vi "niDTS WLAN Tx Test Full Example.vi"() -> ()   [LabVIEW 2014]
uses:
  CommLib/Includes/niDTS Comm INC Telnet Port Parameters.ctl
  CommLib/Includes/niDTS Comm INC CLI Login.ctl
  CommLib/Includes/niDTS Comm INC EXE Port Parameters.ctl
  Includes/niDTS WLAN INC Type.ctl
  OFDM Tx Test/Includes/niDTS WLAN OFDM Tx Test INC Parameters.ctl
  Includes/niDTS WLAN INC OFDM Data Rate.ctl
  Includes/niDTS WLAN INC CH BW DSSS.ctl
  Includes/niDTS WLAN DUT INC Acquisition Parameters.ctl
  Includes/niDTS WLAN INC TXP Measurement Parameters.ctl
  OFDM Tx Test/Includes/niDTS WLAN OFDM Tx Test INC ModAcc Measurement Parameters.ctl
  Includes/niDTS WLAN INC SEM Measurement Parameters.ctl
  Includes/niDTS WLAN INC OBW Measurement Parameters.ctl
  HT Tx Test/Includes/niDTS WLAN HT Tx Test INC Parameters.ctl
  Includes/niDTS WLAN INC CH BW HT.ctl
  Includes/niDTS WLAN INC GI.ctl
  Includes/niDTS WLAN INC FEC Coding.ctl
  VHT Tx Test/Includes/niDTS WLAN VHT Tx Test INC Parameters.ctl
  Includes/niDTS WLAN INC CH BW.ctl
  Tx Test/Includes/niDTS WLAN Tx Test INC Results.ctl
  Tx Test/Includes/niDTS WLAN Tx Test INC MOD EVM Results.ctl
  Tx Test/Includes/Results/niDTS Tx RES INC EVM.ctl
  Tx Test/Includes/niDTS WLAN Tx Test INC TXP Results.ctl
  Tx Test/Includes/niDTS WLAN Tx Test INC TXP Result SINGLE.ctl
  Tx Test/Includes/niDTS WLAN Tx Test INC OBW Results.ctl
  Instrument/INSTR TX/Results/niDTS WLAN INSTR TX INC SEM Results.ctl
  Instrument/INSTR TX/Results/niDTS WLAN INSTR TX INC SEM FSEGemts Results.ctl
  Tx Test/Includes/Results/niDTS Tx RES INC SEM FSEGemts.ctl
  Instrument/INSTR TX/Results/niDTS WLAN INSTR TX INC SEM MARGin Results.ctl
  Tx Test/Includes/Results/niDTS Tx RES INC SEM Margin.ctl
  Instrument/INSTR TX/Results/niDTS WLAN INSTR TX INC OFDM Impairments Results.ctl
  DSSS Tx Test/Includes/niDTS WLAN DSSS Tx Test INC Parameters.ctl
  Includes/niDTS WLAN INC DSSS Data Rate.ctl
  Includes/niDTS WLAN INC Channel DSSS.ctl
  DSSS Tx Test/Includes/niDTS WLAN DSSS Tx Test INC ModAcc Measurement Parameters.ctl
  Includes/niDTS WLAN INC Pulse Shaping Filter Type.ctl
  Includes/niDTS WLAN INC DSSS Power Ramp Parameters.ctl
  Tx Test/Includes/niDTS WLAN Tx Test INC DSSS Results.ctl
  Tx Test/Includes/niDTS WLAN Tx Test INC DSSS MOD EVM Results.ctl
  DSSS Tx Test/Includes/Results/niDTS WLAN DSSS Tx RES EVM ALL.ctl
  DSSS Tx Test/Includes/Results/niDTS WLAN DSSS Tx RES EVM RMS.ctl
  Tx Test/Includes/niDTS WLAN Tx Test INC DSSS MOD Impairments Results.ctl
  DSSS Tx Test/Includes/Results/niDTS WLAN DSSS Tx Impairmentsctl.ctl
  DSSS Tx Test/Includes/Results/niDTS WLAN DSSS Tx PowerRamp.ctl
  TestStand/Station/Objects/SystemDutHandle/niDTS SystemDutHandle.lvclass
  niDTS WLAN.lvlib
  Framework/niDTS Framework.lvlib
  TestStand/niDTS TestStand.lvlib
  Plugins/niBCM4360/niBCM4360.lvlib
  Plugins/niBCM4350/niBCM4350.lvlib
  Plugins/niWTM Loopback/niWTM Loopback.lvlib
  CommLib/niDTS CommLib.lvlib
  Plugins/niBCM4356/niBCM4356.lvlib
  Framework/Logger/Listener/Viewer/niDTS Logger Listener Viewer.lvclass
  Instrument/INSTR TX/niDTS WLAN INSTR TX.lvclass
panel:
  in  "Keep Log Open":bool
  out "DSSS Results":T1 {"OBW"."Stop Frequency (Hz)" format="%#_4p"; "OBW"."Start Frequency (Hz)" format="%#_4p"; "OBW"."OBW (Hz)" format="%#_4p"}
  in  "ResultsIndex":u8=1
  in  "System Configuration XML Path":path=path "C:/Users/Public/Documents/National Instruments/WTM 1.0/System Configurations"
  in  "Socket Index":i32
  out "Results":T16={"Stream ModAcc"={"EVM"={"OFDM EVM Average"=[{"Stream Index"=1, "Packet (dB)"=-38.670074, "Pilot (dB)"=-40.331799, "Data (dB)"=-38.562389}], "OFDM EVM Max"=[{"Stream Index"=1, "Packet (dB)"=-38.670074, "Pilot (dB)"=-40.331799, "Data (dB)"=-38.562389}], "OFDM EVM Min"=[{"Stream Index"=1, "Packet (dB)"=-38.670074, "Pilot (dB)"=-40.331799, "Data (dB)"=-38.562389}]}}, "Channel ModAcc"={"EVM"={"OFDM EVM Average"=[{"Stream Index"=1, "Packet (dB)"=-38.670074, "Pilot (dB)"=-40.331799, "Data (dB)"=-38.562389}], "OFDM EVM Max"=[{"Stream Index"=1, "Packet (dB)"=-38.670074, "Pilot (dB)"=-40.331799, "Data (dB)"=-38.562389}], "OFDM EVM Min"=[{"Stream Index"=1, "Packet (dB)"=-38.670074, "Pilot (dB)"=-40.331799, "Data (dB)"=-38.562389}]}}, "TXP"={"Average"=[{"Chain Index"=1.0, "Average Power (dBm)"=-12.457251, "Peak Power (dBm)"=-4.586085, "Avg Power w Gap (dBm)"=-12.457251}], "Max"=[{"Chain Index"=1.0, "Average Power (dBm)"=-12.457251, "Peak Power (dBm)"=-4.586085, "Avg Power w Gap (dBm)"=-12.457251}], "Min"=[{"Chain Index"=1.0, "Average Power (dBm)"=-12.457251, "Peak Power (dBm)"=-4.586085, "Avg Power w Gap (dBm)"=-12.457251}]}, "OBW"=[{"Chain Index"=1.0, "OBW (Hz)"=17635824.926234, "Start Frequency (Hz)"=5171217983.349262, "Stop Frequency (Hz)"=5188853808.275496}], "SEM Results"={"SEM:FSEGemts"=[], "Margin"=[{"Chain Index"=1, "Worst Case Out Of Band Margin (dB)"=7.826486, "Worst Case Out Of Band Frequency (Hz)"=5191096938.77551, "Violation (%)"=0.0}]}, "OFDM Impairments"={"Average"={"Sample Clock Offset (ppm)"=1.406776, "Carrier Frequency Offset (ppm)"=19.372688, "Avg Rms Com Pilot Error (%)"=0.861502, "Rms Phase Noise (deg)"=0.437853, "ChannelData"=[{"Channel Index"=1, "IQ Imbalance (dB)"=0.0028770000000000002, "Quadrature Skew (deg)"=0.012293, "Carrier Leakage (dB)"=-55.264069, "Timing Skew (s)"=0.0}]}, "Max"={"Sample Clock Offset (ppm)"=1.406776, "Carrier Frequency Offset (ppm)"=19.372688, "Avg Rms Com Pilot Error (%)"=0.861502, "Rms Phase Noise (deg)"=0.437853, "ChannelData"=[{"Channel Index"=1, "IQ Imbalance (dB)"=0.0028770000000000002, "Quadrature Skew (deg)"=0.012293, "Carrier Leakage (dB)"=-55.264069, "Timing Skew (s)"=0.0}]}, "Min"={"Sample Clock Offset (ppm)"=1.406776, "Carrier Frequency Offset (ppm)"=19.372688, "Avg Rms Com Pilot Error (%)"=0.861502, "Rms Phase Noise (deg)"=0.437853, "ChannelData"=[{"Channel Index"=1, "IQ Imbalance (dB)"=0.0028770000000000002, "Quadrature Skew (deg)"=0.012293, "Carrier Leakage (dB)"=-55.264069, "Timing Skew (s)"=0.0}]}}} {"OBW"."Stop Frequency (Hz)" format="%#_4p"; "OBW"."Start Frequency (Hz)" format="%#_4p"; "OBW"."OBW (Hz)" format="%#_4p"}
  out "error out":errorcluster
  in  "DUT Plugin":T20(tab)=enum."BCM4356"
  in  "Interfaces BCM4350":enum32{".EXE", "Telnet"}(tab)
  in  "General Parameters bcm4350 exe":T22={"WLAN"={"Port Parameters EXE"={"Timeout (s)"=5.0}}} caption="General Parameters"
  in  "Socket Parameters bcm4350 exe":cluster{"WLAN":cluster{"IP Address":string}}={"WLAN"={"IP Address"="192.168.1.1"}} caption="Socket Parameters"
  in  "Socket Parameters bcm4350 telnet":cluster{"WLAN":cluster{"IP Address":string}}={"WLAN"={"IP Address"="192.168.1.1"}} caption="Socket Parameters"
  in  "General Parameters bcm4350 telnet":T25={"WLAN"={"Port Parameters Telnet"={"Bytes to Read"=1000, "Line Separator"="\n", "Port Timeout (ms)"=5000, "Read Mode"=enum."normal", "Write Mode"=enum."normal", "Remote Port"=23}, "CLI Login"={"Do Login"=FALSE, "Login Prompt"="", "Password"="", "User Name"=""}}} caption="General Parameters"
  in  "General Parameters 4":T25={"WLAN"={"Port Parameters Telnet"={"Bytes to Read"=1000, "Line Separator"="\n", "Port Timeout (ms)"=5000, "Read Mode"=enum."normal", "Write Mode"=enum."normal", "Remote Port"=23}, "CLI Login"={"Do Login"=TRUE, "Login Prompt"="localhost login: ", "Password"="labview", "User Name"="root"}}} caption="General Parameters"
  in  "Socket Parameters bcm4356":cluster{"WLAN":cluster{"IP Address":string}}[](array[cluster])=[{"WLAN"={"IP Address"="192.168.0.31"}}, {"WLAN"={"IP Address"="192.168.0.32"}}, {"WLAN"={"IP Address"="192.168.0.33"}}, {"WLAN"={"IP Address"="192.168.0.34"}}] caption="Socket Parameters"
  in  "Socket Parameters":T26={"WLAN"={"VISA Resource"="TCPIP0::InstrumentAddress::inst0::INSTR", "PortNames "=["Port0"]}}
  in  "General Parameters":T27={"WLAN"={"Idle Interval (s)"=0.0001, "Payload Length Limit (bytes)"=12000, "Channel Secondary Factor"=enum."0"}} {"WLAN"."Idle Interval (s)" format="%_3p"}
  in  "Test Config":enum32{"DSSS", "OFDM", "HT", "VHT"}(tab)=enum."OFDM"
  in  "DSSS Parameters":T28={"DSSS Data Rate (Mbps)"=enum."1", "Chains"=[TRUE, FALSE, FALSE, FALSE], "Bandwidth (Hz)"=enum."20 MHz", "Channel"=1, "Dut Tx Power  (dBm)"=-20.0, "16 symbols"=TRUE, "Payload Length (bytes)"=1500, "Idle Interval (s)"=0.0001, "External Attenuation (dB)"=[0.0, 0.0, 0.0, 0.0], "Acquisition "={"Acquisition Length Mode"=enum."AUTO", "Acquisition Length (s)"=0.00015, "Auto Level"=FALSE}, "TXP Measurement"={"TXP Power Enable"=TRUE, "TXP Averages"=1}, "ModAcc Measurement"={"ModAcc Enable"=TRUE, "Header Detection"=enum."FIRST", "Averages"=1, "CFO Estimation"=enum."PAMBLE", "DC Offset Compensation"=FALSE, "Chip Start Location"=0, "Max Chips Used"=16, "Pulse Shaping FilterType"=enum."RCOSINE", "Pulse Shaping Filter Coefficient"=0.35, "Equalization"=TRUE, "Phase Tracking"=TRUE}, "SEM Measurement"={"SEM Enable"=TRUE, "SEM Averages"=1, "Auto Span Enable"=TRUE, "Frequency Span (Hz)"=66000000.0, "Measurement Type"=enum."Standard", "Mask Frequencies (Hz)"=[], "Mask Power Offsets (dB)"=[]}, "OBW Measurement"={"OBW Enable"=TRUE, "OBW Averages"=1}, "DSSS Power Ramp"={"Power Ramp Enable"=TRUE, "Averages"=3, "Thresholds"={"Up Low (%)"=10.0, "Down Low (%)"=10.0, "Up High (%)"=90.0, "Down High (%)"=90.0}}} {"DSSS Power Ramp"."Thresholds"."Down High (%)" min=0.0 max=100.0 step=1.0; "DSSS Power Ramp"."Thresholds"."Up High (%)" min=0.0 max=100.0 step=1.0; "DSSS Power Ramp"."Thresholds"."Down Low (%)" min=0.0 max=100.0 step=1.0; "DSSS Power Ramp"."Thresholds"."Up Low (%)" min=0.0 max=100.0 step=1.0; "Acquisition"."Acquisition Length (s)" format="%#_6p"; "SEM Measurement"."Frequency Span (Hz)" format="%#_6p"; "Channel" items=["1"=1, "2"=2, "3"=3, "4"=4, "5"=5, "6"=6, "7"=7, "8"=8, "9"=9, "10"=10, "11"=11, "12"=12, "13"=13, "14"=14]; "Idle Interval (s)" format="%_3p"}
  in  "OFDM Parameters":T39={"OFDM Data Rate (Mbps)"=enum."54", "Chains"=[TRUE, FALSE, FALSE, FALSE], "Bandwidth (Hz)"=enum."20 MHz", "Channel"=36, "Dut Tx Power (dBm)"=-20.0, "16 symbols"=TRUE, "Payload Length (bytes)"=1500, "Idle Interval (s)"=0.0001, "External Attenuation (dB)"=[0.0, 0.0, 0.0, 0.0], "Acquisition "={"Acquisition Length Mode"=enum."AUTO", "Acquisition Length (s)"=0.00015, "Auto Level"=FALSE}, "TXP Measurement"={"TXP Power Enable"=TRUE, "TXP Averages"=1}, "ModAcc Measurement"={"ModAcc Enable"=TRUE, "Header Detection"=enum."FIRST", "Averages"=1, "CFO Estimation"=enum."PAMBLE", "Amplitude Tracking"=FALSE, "Channel Tracking"=FALSE, "Time Tracking"=TRUE, "Phase Tracking"=enum."STANDARD", "Clock Offset Est"=TRUE, "Impairments Est"=TRUE}, "SEM Measurement"={"SEM Enable"=TRUE, "SEM Averages"=1, "Auto Span Enable"=TRUE, "Frequency Span (Hz)"=66000000.0, "Measurement Type"=enum."Standard", "Mask Frequencies (Hz)"=[], "Mask Power Offsets (dB)"=[]}, "OBW Measurement"={"OBW Enable"=TRUE, "OBW Averages"=1}} {"Acquisition"."Acquisition Length (s)" format="%#_6p"; "SEM Measurement"."Frequency Span (Hz)" format="%#_6p"; "Idle Interval (s)" format="%_3p"}
  in  "HT Parameters":T42={"MCS Index"=7, "Chains"=[TRUE, FALSE, FALSE, FALSE], "Bandwidth (Hz)"=enum."20 MHz", "Channel"=36, "Gard Interval"=enum."LONG", "FEC Coding"=enum."LDPC", "Dut Tx Power (dBm)"=10.0, "16 symbols"=TRUE, "Payload Length (bytes)"=1500, "Idle Interval (s)"=0.0001, "External Attenuation (dB)"=[0.0, 0.0, 0.0, 0.0], "Acquisition"={"Acquisition Length Mode"=enum."AUTO", "Acquisition Length (s)"=0.00015, "Auto Level"=FALSE}, "TXP Measurement"={"TXP Power Enable"=TRUE, "TXP Averages"=1}, "ModAcc Measurement"={"ModAcc Enable"=TRUE, "Header Detection"=enum."FIRST", "Averages"=1, "CFO Estimation"=enum."PAMBLE", "Amplitude Tracking"=FALSE, "Channel Tracking"=FALSE, "Time Tracking"=TRUE, "Phase Tracking"=enum."STANDARD", "Clock Offset Est"=TRUE, "Impairments Est"=TRUE}, "SEM Measurement"={"SEM Enable"=TRUE, "SEM Averages"=1, "Auto Span Enable"=TRUE, "Frequency Span (Hz)"=66000000.0, "Measurement Type"=enum."Standard", "Mask Frequencies (Hz)"=[], "Mask Power Offsets (dB)"=[]}, "OBW Measurement"={"OBW Enable"=TRUE, "OBW Averages"=1}} {"Acquisition"."Acquisition Length (s)" format="%#_6p"; "SEM Measurement"."Frequency Span (Hz)" format="%#_6p"; "Idle Interval (s)" format="%_3p"}
  in  "VHT Parameters":T46={"MCS Index"=7, "N Spatial Streams"=1, "Chains"=[TRUE, FALSE, FALSE, FALSE], "Bandwidth (Hz)"=enum."20 MHz", "Channel"=36, "Gard Interval"=enum."LONG", "FEC Coding"=enum."LDPC", "Dut Tx Power (dBm)"=-20.0, "16 symbols"=TRUE, "Payload Length (bytes)"=1500, "Idle Interval (s)"=0.0001, "External Attenuation (dB)"=[0.0, 0.0, 0.0, 0.0], "Acquisition "={"Acquisition Length Mode"=enum."AUTO", "Acquisition Length (s)"=0.00015, "Auto Level"=FALSE}, "TXP Measurement"={"TXP Power Enable"=TRUE, "TXP Averages"=1}, "ModAcc Measurement"={"ModAcc Enable"=TRUE, "Header Detection"=enum."FIRST", "Averages"=1, "CFO Estimation"=enum."PAMBLE", "Amplitude Tracking"=FALSE, "Channel Tracking"=FALSE, "Time Tracking"=TRUE, "Phase Tracking"=enum."STANDARD", "Clock Offset Est"=TRUE, "Impairments Est"=TRUE}, "SEM Measurement"={"SEM Enable"=TRUE, "SEM Averages"=1, "Auto Span Enable"=TRUE, "Frequency Span (Hz)"=66000000.0, "Measurement Type"=enum."Standard", "Mask Frequencies (Hz)"=[], "Mask Power Offsets (dB)"=[]}, "OBW Measurement"={"OBW Enable"=TRUE, "OBW Averages"=1}} {"Acquisition"."Acquisition Length (s)" format="%#_6p"; "SEM Measurement"."Frequency Span (Hz)" format="%#_6p"; "Idle Interval (s)" format="%_3p"}
  out "Results Type":T48=enum."n - MCS7"
  # "No Options"
  # "Note the \\s after login:"
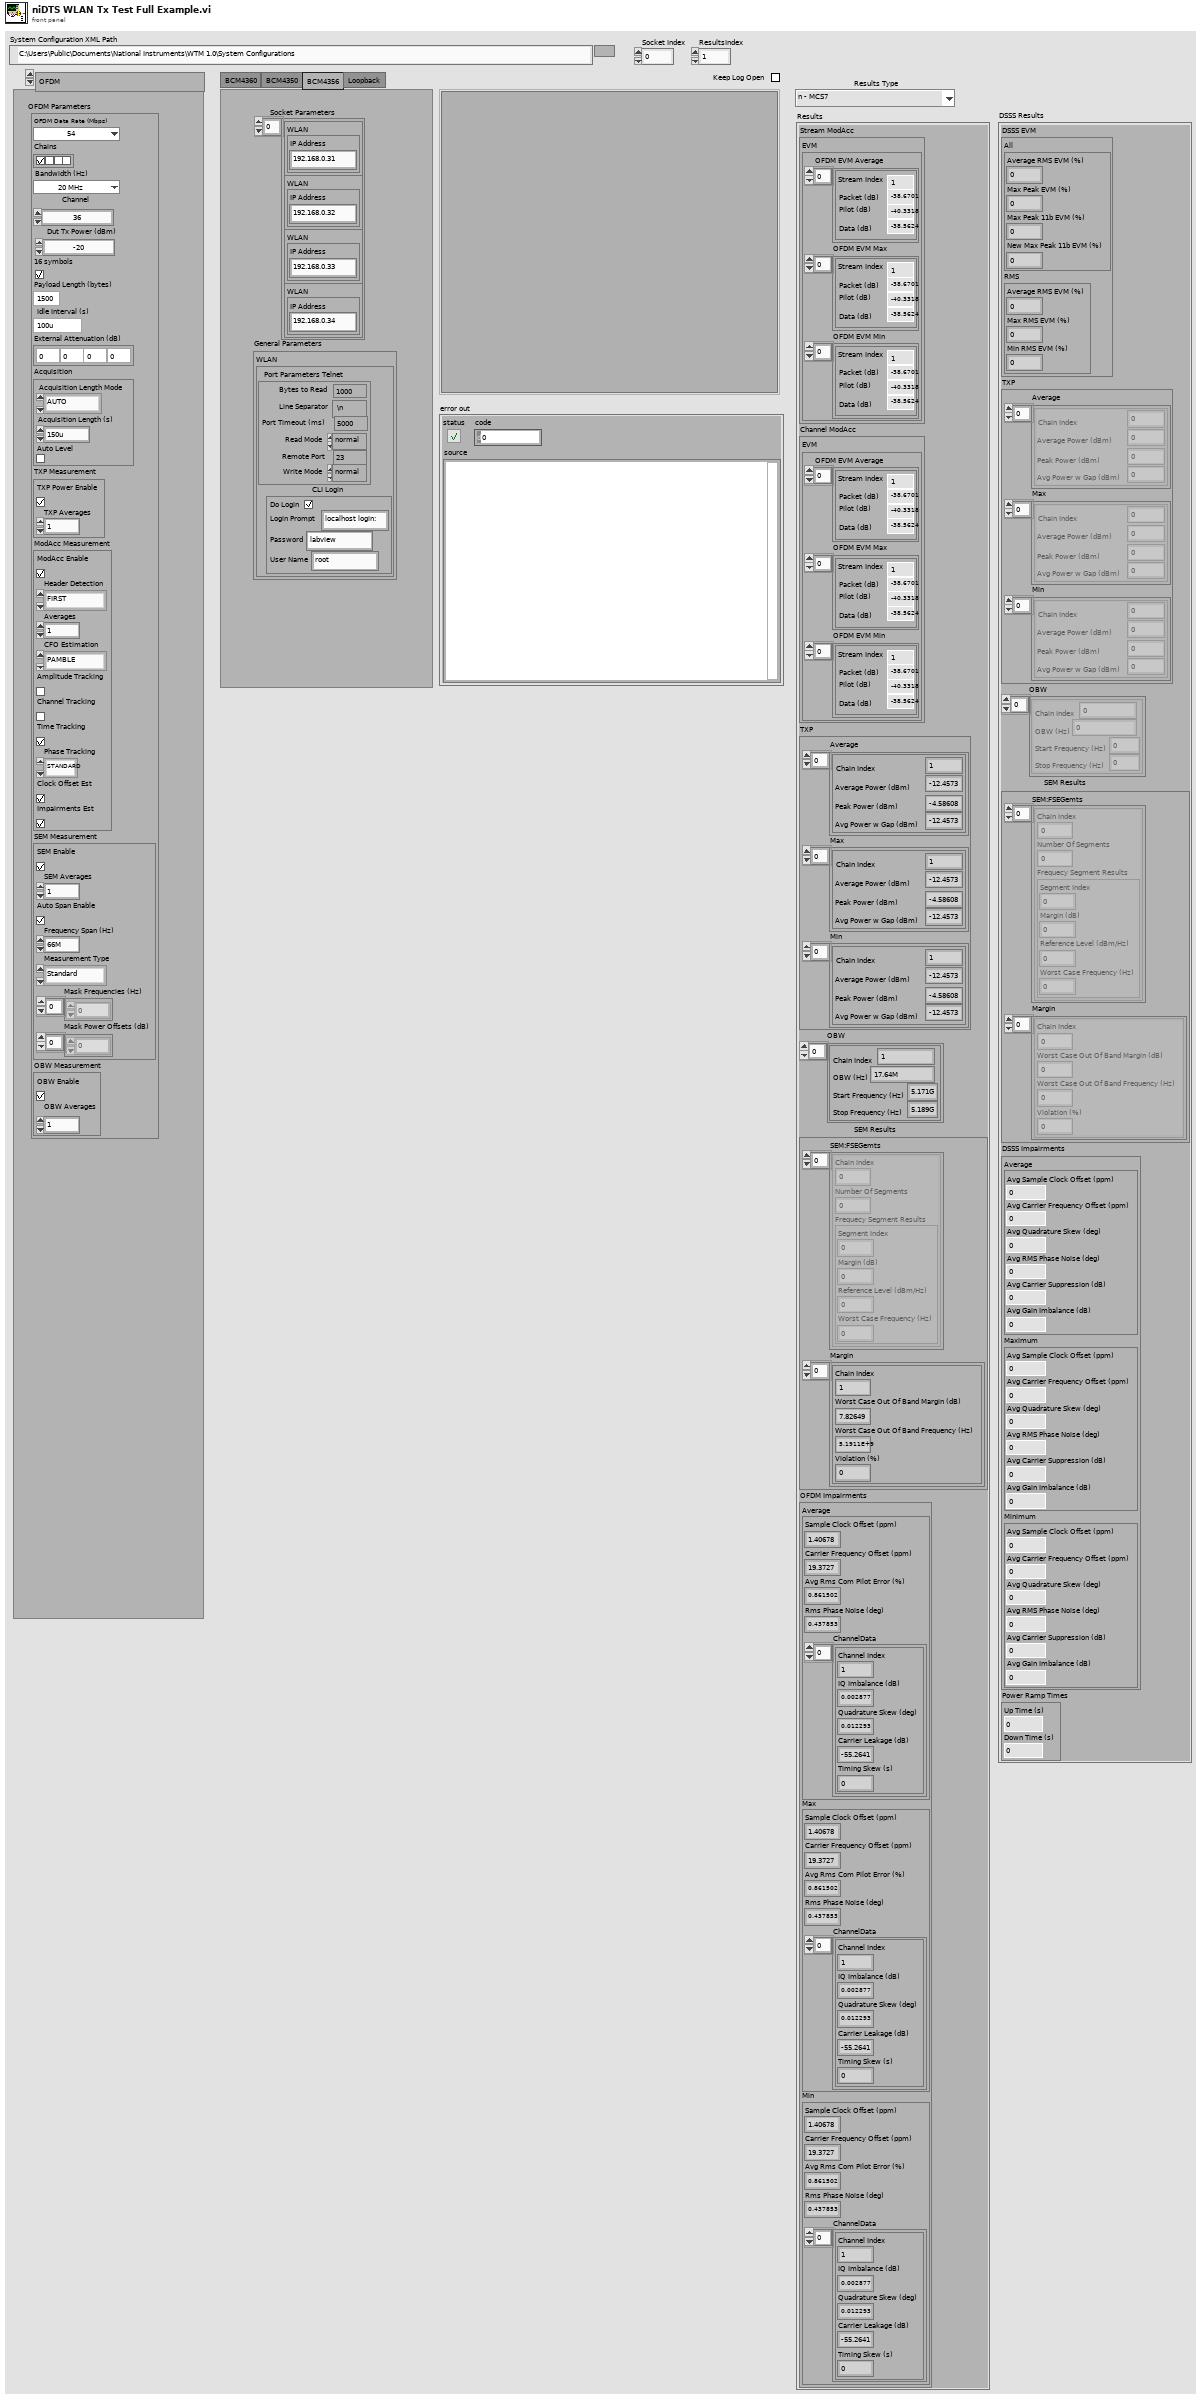
[diagram p1: front panel]
types:
  T1 = typedef "niDTS WLAN.lvlib/niDTS WLAN Tx Test INC DSSS Results.ctl" = cluster{"DSSS EVM":T2, "TXP":T5, "OBW":T7[], "SEM Results":T8, "DSSS Impairments":T13, "Power Ramp Times":T15}
  T2 = typedef "niDTS WLAN.lvlib/niDTS WLAN Tx Test INC DSSS MOD EVM Results.ctl" = cluster{"All":T3, "RMS":T4}
  T3 = typedef "niDTS WLAN.lvlib/niDTS WLAN DSSS Tx RES EVM ALL.ctl" = cluster{"Average RMS EVM (%)":dbl, "Max Peak EVM (%)":dbl, "Max Peak 11b EVM (%)":dbl, "New Max Peak 11b EVM (%)":dbl}
  T4 = typedef "niDTS WLAN.lvlib/niDTS WLAN DSSS Tx RES EVM RMS.ctl" = cluster{"Average RMS EVM (%)":dbl, "Max RMS EVM (%)":dbl, "Min RMS EVM (%)":dbl}
  T5 = typedef "niDTS WLAN.lvlib/niDTS WLAN Tx Test INC TXP Results.ctl" = cluster{"Average":T6[], "Max":T6[], "Min":T6[]}
  T6 = typedef "niDTS WLAN.lvlib/niDTS WLAN Tx Test INC TXP Result SINGLE.ctl" = cluster{"Chain Index":dbl, "Average Power (dBm)":dbl, "Peak Power (dBm)":dbl, "Avg Power w Gap (dBm)":dbl}
  T7 = typedef "niDTS WLAN.lvlib/niDTS WLAN Tx Test INC OBW Results.ctl" = cluster{"Chain Index":dbl, "OBW (Hz)":dbl, "Start Frequency (Hz)":dbl, "Stop Frequency (Hz)":dbl}
  T8 = typedef "niDTS WLAN.lvlib/niDTS WLAN INSTR TX.lvclass/niDTS WLAN INSTR TX INC SEM Results.ctl" = cluster{"SEM:FSEGemts":T9, "Margin":T11}
  T9 = typedef "niDTS WLAN.lvlib/niDTS WLAN INSTR TX.lvclass/niDTS WLAN INSTR TX INC SEM FSEGemts Results.ctl" = T10[]
  T10 = typedef "niDTS WLAN.lvlib/niDTS Tx RES INC SEM FSEGemts.ctl" = cluster{"Chain Index":i32, "Number Of Segments":i32, "Frequecy Segment Results":cluster{"Segment Index":i32, "Margin (dB)":dbl, "Reference Level (dBm/Hz)":dbl, "Worst Case Frequency (Hz)":dbl}}
  T11 = typedef "niDTS WLAN.lvlib/niDTS WLAN INSTR TX.lvclass/niDTS WLAN INSTR TX INC SEM MARGin Results.ctl" = T12[]
  T12 = typedef "niDTS WLAN.lvlib/niDTS Tx RES INC SEM Margin.ctl" = cluster{"Chain Index":i32, "Worst Case Out Of Band Margin (dB)":dbl, "Worst Case Out Of Band Frequency (Hz)":dbl, "Violation (%)":dbl}
  T13 = typedef "niDTS WLAN.lvlib/niDTS WLAN Tx Test INC DSSS MOD Impairments Results.ctl" = cluster{"Average":T14, "Maximum":T14, "Minimum":T14}
  T14 = typedef "niDTS WLAN.lvlib/niDTS WLAN DSSS Tx Impairmentsctl.ctl" = cluster{"Avg Sample Clock Offset (ppm)":dbl, "Avg Carrier Frequency Offset (ppm)":dbl, "Avg Quadrature Skew (deg)":dbl, "Avg RMS Phase Noise (deg)":dbl, "Avg Carrier Suppression (dB)":dbl, "Avg Gain Imbalance (dB)":dbl}
  T15 = typedef "niDTS WLAN.lvlib/niDTS WLAN DSSS Tx PowerRamp.ctl" = cluster{"Up Time (s)":dbl, "Down Time (s)":dbl}
  T16 = typedef "niDTS WLAN.lvlib/niDTS WLAN Tx Test INC Results.ctl" = cluster{"Stream ModAcc":T17, "Channel ModAcc":T17, "TXP":T5, "OBW":T7[], "SEM Results":T8, "OFDM Impairments":T19}
  T17 = typedef "niDTS WLAN.lvlib/niDTS WLAN Tx Test INC MOD EVM Results.ctl" = cluster{"EVM":cluster{"OFDM EVM Average":T18[], "OFDM EVM Max":T18[], "OFDM EVM Min":T18[]}}
  T18 = typedef "niDTS WLAN.lvlib/niDTS Tx RES INC EVM.ctl" = cluster{"Stream Index":i32, "Packet (dB)":dbl, "Pilot (dB)":dbl, "Data (dB)":dbl}
  T19 = typedef "niDTS WLAN.lvlib/niDTS WLAN INSTR TX.lvclass/niDTS WLAN INSTR TX INC OFDM Impairments Results.ctl" = cluster{"Average":cluster{"Sample Clock Offset (ppm)":dbl, "Carrier Frequency Offset (ppm)":dbl, "Avg Rms Com Pilot Error (%)":dbl, "Rms Phase Noise (deg)":dbl, "ChannelData":cluster{"Channel Index":i32, "IQ Imbalance (dB)":dbl, "Quadrature Skew (deg)":dbl, "Carrier Leakage (dB)":dbl, "Timing Skew (s)":dbl}[]}, "Max":cluster{"Sample Clock Offset (ppm)":dbl, "Carrier Frequency Offset (ppm)":dbl, "Avg Rms Com Pilot Error (%)":dbl, "Rms Phase Noise (deg)":dbl, "ChannelData":cluster{"Channel Index":i32, "IQ Imbalance (dB)":dbl, "Quadrature Skew (deg)":dbl, "Carrier Leakage (dB)":dbl, "Timing Skew (s)":dbl}[]}, "Min":cluster{"Sample Clock Offset (ppm)":dbl, "Carrier Frequency Offset (ppm)":dbl, "Avg Rms Com Pilot Error (%)":dbl, "Rms Phase Noise (deg)":dbl, "ChannelData":cluster{"Channel Index":i32, "IQ Imbalance (dB)":dbl, "Quadrature Skew (deg)":dbl, "Carrier Leakage (dB)":dbl, "Timing Skew (s)":dbl}[]}}
  T20 = enum32{"BCM4360", "BCM4350", "BCM4356", "Loopback"}
  T21 = typedef "niDTS CommLib.lvlib/niDTS Comm INC EXE Port Parameters.ctl" = cluster{"Timeout (s)":dbl}
  T22 = cluster{"WLAN":cluster{"Port Parameters EXE":T21}}
  T23 = typedef "niDTS CommLib.lvlib/niDTS Comm INC Telnet Port Parameters.ctl" = cluster{"Bytes to Read":i32, "Line Separator":string, "Port Timeout (ms)":i32, "Read Mode":enum16{"normal", "line", "buffered"}, "Write Mode":enum16{"normal", "line", "buffered"}, "Remote Port":u16}
  T24 = typedef "niDTS CommLib.lvlib/niDTS Comm INC CLI Login.ctl" = cluster{"Do Login":bool, "Login Prompt":string, "Password":string, "User Name":string}
  T25 = cluster{"WLAN":cluster{"Port Parameters Telnet":T23, "CLI Login":T24}}
  T26 = cluster{"WLAN":cluster{"VISA Resource":string, "PortNames ":string[]}}
  T27 = cluster{"WLAN":cluster{"Idle Interval (s)":dbl, "Payload Length Limit (bytes)":i32, "Channel Secondary Factor":enum16{"-1", "1", "0"}}}
  T28 = typedef "niDTS WLAN.lvlib/niDTS WLAN DSSS Tx Test INC Parameters.ctl" = cluster{"DSSS Data Rate (Mbps)":T29, "Chains":bool[], "Bandwidth (Hz)":T30, "Channel":T31, "Dut Tx Power  (dBm)":dbl, "16 symbols":bool, "Payload Length (bytes)":i32, "Idle Interval (s)":dbl, "External Attenuation (dB)":dbl[], "Acquisition ":T32, "TXP Measurement":T33, "ModAcc Measurement":T34, "SEM Measurement":T36, "OBW Measurement":T37, "DSSS Power Ramp":T38}
  T29 = typedef "niDTS WLAN.lvlib/niDTS WLAN INC DSSS Data Rate.ctl" = enum16{"1", "2", "5.5", "11"}
  T30 = typedef "niDTS WLAN.lvlib/niDTS WLAN INC CH BW DSSS.ctl" = enum16{"20 MHz"}
  T31 = typedef "niDTS WLAN.lvlib/niDTS WLAN INC Channel DSSS.ctl" = i8
  T32 = typedef "niDTS WLAN.lvlib/niDTS WLAN DUT INC Acquisition Parameters.ctl" = cluster{"Acquisition Length Mode":enum16{"AUTO", "MANUAL"}, "Acquisition Length (s)":dbl, "Auto Level":bool}
  T33 = typedef "niDTS WLAN.lvlib/niDTS WLAN INC TXP Measurement Parameters.ctl" = cluster{"TXP Power Enable":bool, "TXP Averages":i32}
  T34 = typedef "niDTS WLAN.lvlib/niDTS WLAN DSSS Tx Test INC ModAcc Measurement Parameters.ctl" = cluster{"ModAcc Enable":bool, "Header Detection":enum16{"MANUAL", "FIRST", "ALL"}, "Averages":i32, "CFO Estimation":enum16{"PAMBLE", "PDATA"}, "DC Offset Compensation":bool, "Chip Start Location":i16, "Max Chips Used":i16, "Pulse Shaping FilterType":T35, "Pulse Shaping Filter Coefficient":dbl, "Equalization":bool, "Phase Tracking":bool}
  T35 = typedef "niDTS WLAN.lvlib/niDTS WLAN INC Pulse Shaping Filter Type.ctl" = enum16{"NONE", "RCOSINE", "RRCOSINE", "GAUSSIAN"}
  T36 = typedef "niDTS WLAN.lvlib/niDTS WLAN INC SEM Measurement Parameters.ctl" = cluster{"SEM Enable":bool, "SEM Averages":i32, "Auto Span Enable":bool, "Frequency Span (Hz)":dbl, "Measurement Type":enum16{"Standard", "Legacy", "Custom"}, "Mask Frequencies (Hz)":dbl[], "Mask Power Offsets (dB)":dbl[]}
  T37 = typedef "niDTS WLAN.lvlib/niDTS WLAN INC OBW Measurement Parameters.ctl" = cluster{"OBW Enable":bool, "OBW Averages":i32}
  T38 = typedef "niDTS WLAN.lvlib/niDTS WLAN INC DSSS Power Ramp Parameters.ctl" = cluster{"Power Ramp Enable":bool, "Averages":i32, "Thresholds":cluster{"Up Low (%)":dbl, "Down Low (%)":dbl, "Up High (%)":dbl, "Down High (%)":dbl}}
  T39 = typedef "niDTS WLAN.lvlib/niDTS WLAN OFDM Tx Test INC Parameters.ctl" = cluster{"OFDM Data Rate (Mbps)":T40, "Chains":bool[], "Bandwidth (Hz)":T30, "Channel":i32, "Dut Tx Power (dBm)":dbl, "16 symbols":bool, "Payload Length (bytes)":i32, "Idle Interval (s)":dbl, "External Attenuation (dB)":dbl[], "Acquisition ":T32, "TXP Measurement":T33, "ModAcc Measurement":T41, "SEM Measurement":T36, "OBW Measurement":T37}
  T40 = typedef "niDTS WLAN.lvlib/niDTS WLAN INC OFDM Data Rate.ctl" = enum16{"6", "9", "12", "18", "24", "36", "48", "54"}
  T41 = typedef "niDTS WLAN.lvlib/niDTS WLAN OFDM Tx Test INC ModAcc Measurement Parameters.ctl" = cluster{"ModAcc Enable":bool, "Header Detection":enum16{"MANUAL", "FIRST", "ALL"}, "Averages":i32, "CFO Estimation":enum16{"PAMBLE", "PDATA"}, "Amplitude Tracking":bool, "Channel Tracking":bool, "Time Tracking":bool, "Phase Tracking":enum16{"NONE", "STANDARD", "CSF", "INSTANT"}, "Clock Offset Est":bool, "Impairments Est":bool}
  T42 = typedef "niDTS WLAN.lvlib/niDTS WLAN HT Tx Test INC Parameters.ctl" = cluster{"MCS Index":i32, "Chains":bool[], "Bandwidth (Hz)":T43, "Channel":i32, "Gard Interval":T44, "FEC Coding":T45, "Dut Tx Power (dBm)":dbl, "16 symbols":bool, "Payload Length (bytes)":i32, "Idle Interval (s)":dbl, "External Attenuation (dB)":dbl[], "Acquisition":T32, "TXP Measurement":T33, "ModAcc Measurement":T41, "SEM Measurement":T36, "OBW Measurement":T37}
  T43 = typedef "niDTS WLAN.lvlib/niDTS WLAN INC CH BW HT.ctl" = enum16{"20 MHz", "40 MHz"}
  T44 = typedef "niDTS WLAN.lvlib/niDTS WLAN INC GI.ctl" = enum16{"LONG", "SHORT"}
  T45 = typedef "niDTS WLAN.lvlib/niDTS WLAN INC FEC Coding.ctl" = enum16{"BCC", "LDPC"}
  T46 = typedef "niDTS WLAN.lvlib/niDTS WLAN VHT Tx Test INC Parameters.ctl" = cluster{"MCS Index":i32, "N Spatial Streams":i32, "Chains":bool[], "Bandwidth (Hz)":T47, "Channel":i32, "Gard Interval":T44, "FEC Coding":T45, "Dut Tx Power (dBm)":dbl, "16 symbols":bool, "Payload Length (bytes)":i32, "Idle Interval (s)":dbl, "External Attenuation (dB)":dbl[], "Acquisition ":T32, "TXP Measurement":T33, "ModAcc Measurement":T41, "SEM Measurement":T36, "OBW Measurement":T37}
  T47 = typedef "niDTS WLAN.lvlib/niDTS WLAN INC CH BW.ctl" = enum16{"20 MHz", "40 MHz", "80 MHz", "160 MHz"}
  T48 = typedef "niDTS WLAN.lvlib/niDTS WLAN INC Type.ctl" = enum16{"b - 1 Mbps", "b - 2 Mbps", "b - 5.5 Mbps", "b - 11 Mbps", "ag - 6 Mbps", "ag - 9 Mbps", "ag - 12 Mbps", "ag - 18 Mbps", "ag - 24 Mbps", "ag - 36 Mbps", "ag - 48 Mbps", "ag - 54 Mbps", "n - MCS0", "n - MCS1", "n - MCS2", "n - MCS3", "n - MCS4", "n - MCS5", "n - MCS6", "n - MCS7", "n - MCS8", "n - MCS9", "n - MCS10", "n - MCS11", "n - MCS12", "n - MCS13", "n - MCS14", "n - MCS15", "n - MCS16", "n - MCS17", "n - MCS18", "n - MCS19", "n - MCS20", "n - MCS21", "n - MCS22", "n - MCS23", "n - MCS24", "n - MCS25", "n - MCS26", "n - MCS27", "n - MCS28", "n - MCS29", "n - MCS30", "n - MCS31", "ac - MCS0 -1", "ac - MCS1 -1", "ac - MCS2 -1", "ac - MCS3 -1", "ac - MCS4 -1", "ac - MCS5 -1", "ac - MCS6 -1", "ac - MCS7 -1", "ac - MCS8 -1", "ac - MCS9 -1", "ac - MCS0 -2", "ac - MCS1 -2", "ac - MCS2 -2", "ac - MCS3 -2", "ac - MCS4 -2", "ac - MCS5 -2", "ac - MCS6 -2", "ac - MCS7 -2", "ac - MCS8 -2", "ac - MCS9 -2", "ac - MCS0 -3", "ac - MCS1 -3", "ac - MCS2 -3", "ac - MCS3 -3", "ac - MCS4 -3", "ac - MCS5 -3", "ac - MCS6 -3", "ac - MCS7 -3", "ac - MCS8 -3", "ac - MCS9 -3", "ac - MCS0 -4", "ac - MCS1 -4", "ac - MCS2 -4", "ac - MCS3 -4", "ac - MCS4 -4", "ac - MCS5 -4", "ac - MCS6 -4", "ac - MCS7 -4", "ac - MCS8 -4", "ac - MCS9 -4"}
  T49 = typedef "niDTS Framework.lvlib/niDTS Logger INC Handle.ctl" = refnum<data-value>
  T50 = cluster{"WLAN":cluster{"VISA Resource":string, "PortNames ":string[]}, "Bluetooth":cluster{"VISA Resource":string, "PortNames ":string[]}, "GNSS":cluster{"VISA Resource":string, "PortNames ":string[]}}
  T51 = typedef "niDTS TestStand.lvlib/niDTS SystemDutHandle.lvclass/niDTS SystemDutHandle INC SystemDutHandles.ctl" = refnum<class "niDTS SystemDutHandle.lvclass">[]
  T52 = cluster{"VISA Resource":string, "PortNames ":string[]}
  T53 = typedef "niDTS Framework.lvlib/niDTS Dut INC Handle.ctl" = refnum<data-value>
  T54 = typedef "niDTS WLAN.lvlib/niDTS WLAN Tx Test INC Handle.ctl" = refnum<data-value>
  T55 = typedef "niDTS WLAN.lvlib/niDTS WLAN Tx Test INC Parameters.ctl" = cluster{"Standard":T56, "DSSS Data Rate (Mbps)":T29, "OFDM Data Rate (Mbps)":T40, "MCS Index":i32, "N spatial streams":i32, "Chains":bool[], "BandWidth (Hz)":T47, "Channel":i32, "Gard Interval":T44, "FEC Coding":T45, "Dut Tx Power":dbl, "16 symbols":bool, "payload length bytes":i32, "idle interval":dbl, "External Attenuation":dbl[], "Acquisition Parameters ":T32, "TXP Measurement Parameters":T33, "ModAcc Measurement Paramaters":T57, "ModAcc DSSS Paramaters":T58, "SEM Measurement Parameters":T36, "OBW Measurement Parameters":T37, "DSSS Power Ramp":T38, "Enable Traces":bool}
  T56 = typedef "niDTS WLAN.lvlib/niDTS WLAN INC Standard.ctl" = enum16{"802.11 b DSSS", "802.11 a/g OFDM", "802.11 n HT", "802.11 ac VHT"}
  T57 = typedef "niDTS WLAN.lvlib/niDTS WLAN INC ModAcc Measurement Parameters.ctl" = cluster{"ModAcc Enable":bool, "Header Detection":enum16{"MANUAL", "FIRST", "ALL"}, "Averages":i32, "Amplitude Tracking":bool, "Channel Tracking":bool, "Time Tracking":bool, "Phase Tracking":enum16{"NONE", "STANDARD", "CSF", "INSTANT"}, "Clock Offset Est":bool, "Impairments Est":bool, "CFO Estimation":enum16{"PAMBLE", "PDATA"}}
  T58 = typedef "niDTS WLAN.lvlib/niDTS WLAN INC DSSS ModAcc Measurement Parameters.ctl" = cluster{"DC Offset Compensation":bool, "Equalization":bool, "Phase Tracking":bool, "Chip Start Location":i16, "Max Chips Used":i16, "Pulse Shaping FilterType":T35, "Pulse Shaping Filter Coefficient":dbl}
  T59 = typedef "niDTS WLAN.lvlib/niDTS WLAN DUT INC Parameters.ctl" = cluster{"WLAN Type":T48, "Bandwidth (Hz)":T47, "Channel":i32, "Guard Interval":T44, "FEC Coding":T45, "Power (dBm)":dbl, "Payload Length (bytes)":i32, "16 Symbols":bool, "Chains":bool[]}
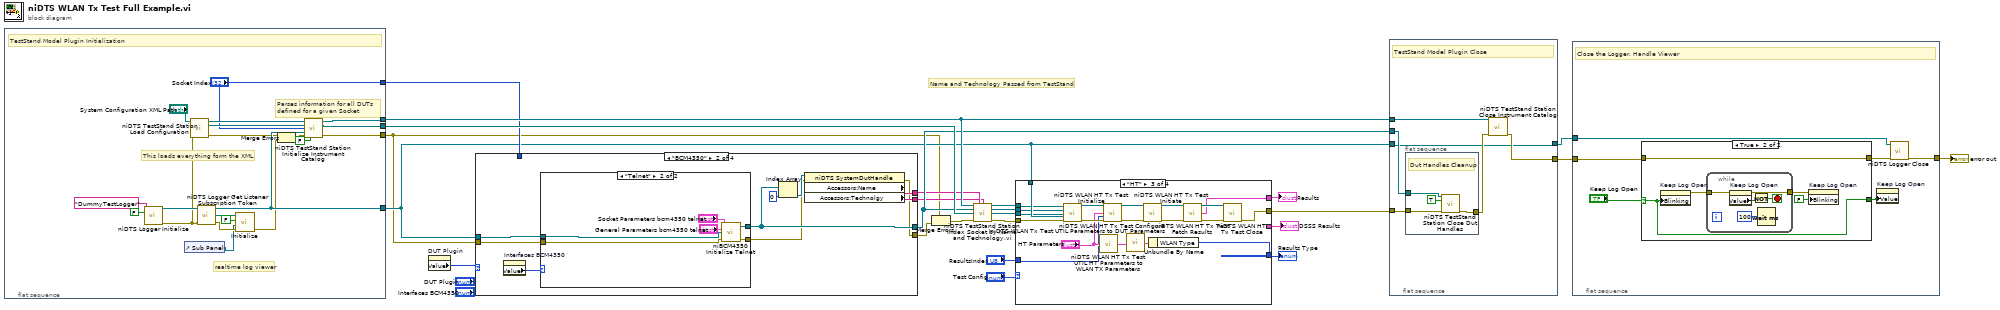
[diagram p0: block diagram]
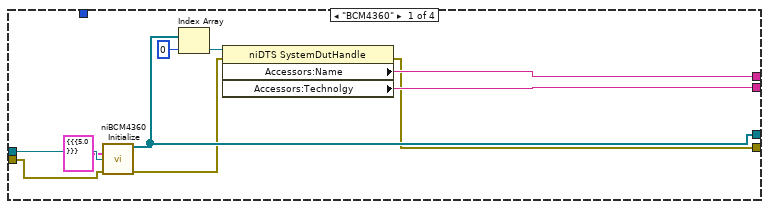
[diagram p3: hidden frame]
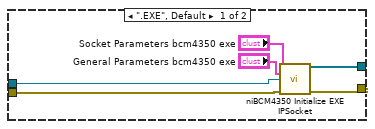
[diagram p4: hidden frame]
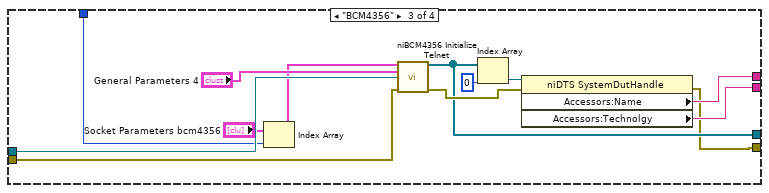
[diagram p5: hidden frame]
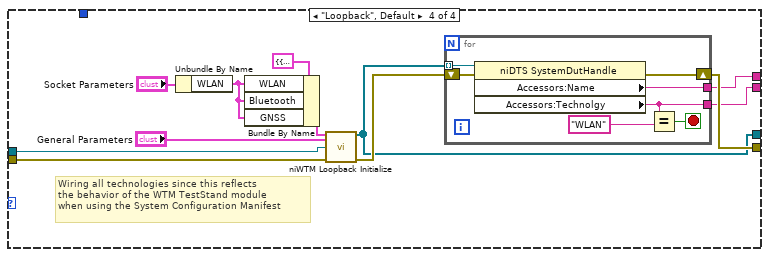
[diagram p6: hidden frame]
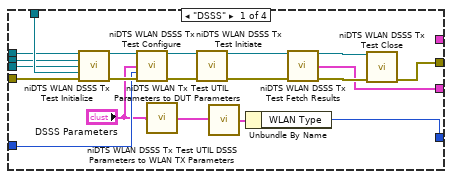
[diagram p7: hidden frame]
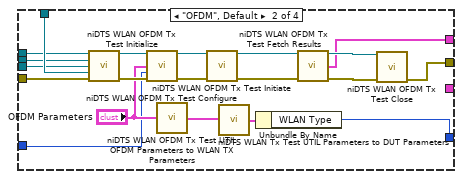
[diagram p8: hidden frame]
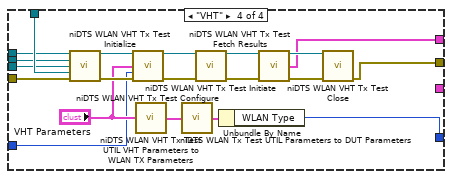
[diagram p9: hidden frame]
diagram:
  # "Name and Technology Passed from TestStand"
  n1 = flat-sequence {
    tunnel: [w38] -> w18
    tunnel: [w39] -> w19
    tunnel: [w37] -> w1
    tunnel: [w28] -> w2
    tunnel: ["Socket Index"] -> w7
    frame #0 {
      # "realtime log viewer"
      # "Parses information for all DUTs defined for a given Socket"
      # "This loads everything form the XML"
      # "TestStand Model Plugin Initialization"
      n2 = call "niDTS Logger Initialize.vi"("Session Name ()"="DummyTestLogger", "Log to File"=FALSE) -> ("Logger Handle out"=w30:T49, "error out"=w29:errorcluster)  [unwired: 12 in]
      n3 = control-ref of="Sub Panel"() -> (w31:refnum<vi>)
      n4 = call "niDTS TestStand Station Load Configuration.vi"("System Configuration XML Path"="System Configuration XML Path", "error in (no error)"=w29) -> ("All System Hardware"=w40:refnum<class "niDTS SystemHardware.lvclass">, "All DUT Definitions"=w42:refnum<class "niDTS SystemDut.lvclass">[], "error out"=w26:errorcluster)  [unwired: 11 in]
      n5 = call "niDTS Logger Get Listener Subscription Token.vi"("Logger Handle in"=w30, "error in (no error)"=w29) -> ("Logger Handle out"=w28:T49, "Listener Subscription Token"=w34:refnum<class "niDTS Logger Listener Subscription Token.lvclass">, "error out"=w33:errorcluster)  [unwired: 11 in]
      n6 = call "Initialize.vi"("error in (no error)"=w33, "SubPanel Reference"=w31, "Open Viewer?"=FALSE, "Listener Subscription Token"=w34) -> ("error out"=w25:errorcluster)  [unwired: 6 in, 1 out]
      n7 = Merge Errors(w26, w25) -> (w27:errorcluster)
      n8 = call "niDTS TestStand Station Initialize Instrument Catalog.vi"("All System Hardware"=w40, "All DUT Definitions"=w42, "Socket Index"="Socket Index", "Logger Handle"=w28, "error in (no error)"=w27, "Simulation Mode (F)"=FALSE) -> ("Socket Instrument Catalog"=w39:refnum<class "niDTS SystemInstrCatalog.lvclass">, "Socket DUT Definitions"=w38:refnum<class "niDTS SystemDut.lvclass">[], "error out"=w37:errorcluster)  [unwired: 7 in]
    }
  }
  n9 = property on="DUT Plugin" class="TabCtl (strict)"() -> ("Value"=w22:T20)  [unwired: 2 in, 2 out]
  n10 = case shown="\"BCM4350\"" w22 {
    tunnel: [w46 w56 w82 w93] -> w20
    tunnel: w2 -> [w54 w64 w81 w101]
    tunnel: [w48 w60 w83 w90] -> w12
    tunnel: [w50 w59 w85 w92] -> w11
    tunnel: [w49 w58 w84 w91] -> w10
    tunnel: w7 -> [_ _ w79 _]
    tunnel: w1 -> [w45 w55 w77 w95]
    frame "BCM4360" {
      n11 = call "niBCM4360 Initialize.vi"("General Parameters"=T22 {"WLAN"={"Port Parameters EXE"={"Timeout (s)"=5.0}}}, "Logger"=w54, "error in (no error)"=w45) -> ("Dut Technology Handles"=w48:T51, "error out"=w47:errorcluster)  [unwired: 11 in]
      n12 = Index Array(array=w48, index=0) -> (element=w51:refnum<class "niDTS SystemDutHandle.lvclass">)
      n13 = property class="niDTS SystemDutHandle"(reference=w51, error in=w47) -> (error out=w46:errorcluster, "Accessors:Name"=w50:string, "Accessors:Technolgy"=w49:string)  [unwired: 1 out]
    }
    frame "BCM4350" {
      n14 = property on="Interfaces BCM4350" class="TabCtl (strict)"() -> ("Value"=w63:enum32{".EXE", "Telnet"})  [unwired: 2 in, 2 out]
      n15 = case shown="\"Telnet\"" w63 {
        tunnel: [w69 w76] -> w57
        tunnel: w64 -> [w68 w72]
        tunnel: [w70 w75] -> w60
        tunnel: w55 -> [w65 w71]
        frame ".EXE", Default {
          n16 = call "niBCM4350 Initialize EXE IPSocket.vi"("Socket Parameters"="Socket Parameters bcm4350 exe", "General Parameters"="General Parameters bcm4350 exe", "Logger"=w68, "error in (no error)"=w65) -> ("Dut Technology Handles 2"=w70:T51, "error out"=w69:errorcluster)  [unwired: 10 in]
        }
        frame "Telnet" {
          n17 = call "niBCM4350 Initialize Telnet.vi"("Socket Parameters"="Socket Parameters bcm4350 telnet", "General Parameters"="General Parameters bcm4350 telnet", "Logger"=w72, "error in (no error)"=w71) -> ("Dut Technology Handles"=w75:T51, "error out"=w76:errorcluster)  [unwired: 10 in]
        }
      }
      n18 = Index Array(array=w60, index=0) -> (element=w61:refnum<class "niDTS SystemDutHandle.lvclass">)
      n19 = property class="niDTS SystemDutHandle"(reference=w61, error in=w57) -> (error out=w56:errorcluster, "Accessors:Name"=w59:string, "Accessors:Technolgy"=w58:string)  [unwired: 1 out]
    }
    frame "BCM4356" {
      n20 = Index Array(array="Socket Parameters bcm4356", index=w79) -> (element=w78:cluster{"WLAN":cluster{"IP Address":string}})
      n21 = call "niBCM4356 Initialize Telnet.vi"("Socket Parameters"=w78, "General Parameters"="General Parameters 4", "Logger"=w81, "error in (no error)"=w77) -> ("Dut Technology Handles"=w83:T51, "error out"=w86:errorcluster)  [unwired: 10 in]
      n22 = Index Array(array=w83, index=0) -> (element=w87:refnum<class "niDTS SystemDutHandle.lvclass">)
      n23 = property class="niDTS SystemDutHandle"(reference=w87, error in=w86) -> (error out=w82:errorcluster, "Accessors:Name"=w85:string, "Accessors:Technolgy"=w84:string)  [unwired: 1 out]
    }
    frame "Loopback", Default {
      # "Wiring all technologies since this reflects \nthe behavior of the WTM TestStand module \nwhen using the System Configuration Manifest"
      n24 = Unbundle By Name("Socket Parameters") -> ("WLAN"=w97:T52)
      n25 = Bundle By Name(cluster=T50 {"WLAN"={"VISA Resource"="TCPIP0::InstrumentAddress::inst0::INSTR", "PortNames "=["Port0"]}, "Bluetooth"={"VISA Resource"="TCPIP0::InstrumentAddress::inst0::INSTR", "PortNames "=["Port0"]}, "GNSS"={"VISA Resource"="TCPIP0::InstrumentAddress::inst0::INSTR", "PortNames "=["Port0"]}} ("Socket Parameters"), "WLAN"=w97, "Bluetooth"=w97, "GNSS"=w97) -> (w96:T50)
      n26 = call "niWTM Loopback Initialize.vi"("Socket Parameters"=w96, "General Parameters"="General Parameters", "Logger"=w101, "error in (no error)"=w95) -> ("Dut Technology Handles"=w90:T51, "error out"=w94:errorcluster)  [unwired: 10 in]
      n27 = for {
        tunnel: [w103] -> w91
        tunnel: [w106] -> w92
        shift-right: [w107] -> w93
        shift-left: w94 -> [w108]
        tunnel: w90 -> [w105] mode=indexing
        stop <- w102 stop-if-true
        n28 = property class="niDTS SystemDutHandle"(reference=w105, error in=w108) -> (error out=w107:errorcluster, "Accessors:Name"=w106:string, "Accessors:Technolgy"=w103:string)  [unwired: 1 out]
        n29 = Equal?(x=w103, y="WLAN") -> (x = y?=w102:bool)
      }
    }
  }
  n30 = Merge Errors(w1, w20) -> (w17:errorcluster)
  n31 = call "niDTS TestStand Station Index Socket by Name and Technology,vi.vi"("niDTS SystemInstrCatalog in"=w19, "Name"=w11, "Technology"=w10, "System Dut Handles"=w12, "Socket DUT Definitions"=w18, "error in (no error)"=w17) -> ("Dut Handle"=w16:T53, "SystemTechnologyCatalog"=w15:refnum<class "niDTS SystemTechnologyCatalog.lvclass">, "Specific Socket/Tech DUT Definition"=w14:refnum<class "niDTS SystemDut.lvclass">, "error out"=w13:errorcluster)  [unwired: 6 in]
  n32 = case shown="\"HT\"" "Test Config" {
    tunnel: [w127 w147 w157 w176] -> w23
    tunnel: [w118 w138 w156 w181] -> w21
    tunnel: w13 -> [w117 w136 w159 w182]
    tunnel: w2 -> [w115 w134 w154 w175]
    tunnel: w16 -> [w114 w133 w153 w173]
    tunnel: w15 -> [w113 w132 w152 w172]
    tunnel: w14 -> [w112 w131 w151 w171]
    tunnel: [_ w130 w150 w170] -> w9
    tunnel: "ResultsIndex" -> [w111 w129 w149 w169]
    tunnel: [w109 _ _ _] -> w6
    frame "DSSS" {
      n33 = call "niDTS WLAN DSSS Tx Test Initialize.vi"("Dut Reference"=w114, "SystemTechnologyCatalog"=w113, "SystemDut"=w112, "Logger Reference"=w115, "error in (no error)"=w117) -> ("OFDM Tx Test Out"=w126:T54, "error out"=w125:errorcluster)  [unwired: 8 in, 1 out]
      n34 = call "niDTS WLAN DSSS Tx Test Configure.vi"("Dummy Test Handle in"=w126, "Cluster"="DSSS Parameters", "ResultsIndex"=w111, "error in (no error)"=w125) -> ("Dummy Test Handle out"=w124:T54, "error out"=w123:errorcluster)  [unwired: 10 in]
      n35 = call "niDTS WLAN DSSS Tx Test UTIL DSSS Parameters to WLAN TX Parameters.vi"("DSSS Parameters"="DSSS Parameters") -> ("WLAN Tx Parameters"=w116:T55)  [unwired: 14 in]
      n36 = call "niDTS WLAN DSSS Tx Test Initiate.vi"("Dummy Test Handle in"=w124, "error in (no error)"=w123) -> ("Dummy Test Handle out"=w122:T54, "error out"=w121:errorcluster)  [unwired: 12 in]
      n37 = call "niDTS WLAN Tx Test UTIL Parameters to DUT Parameters.vi"("Parameters"=w116) -> ("TV Parameters(DataType)"=w128:T59)  [unwired: 14 in]
      n38 = Unbundle By Name(w128) -> ("WLAN Type"=w127:T48)
      n39 = call "niDTS WLAN DSSS Tx Test Fetch Results.vi"("Dummy Test Handle in"=w122, "error in (no error)"=w121) -> ("Dummy Test Handle out"=w120:T54, "Results"=w109:T1, "error out"=w119:errorcluster)  [unwired: 11 in]
      n40 = call "niDTS WLAN DSSS Tx Test Close.vi"("Dummy Test Handle in"=w120, "error in (no error)"=w119) -> ("error out"=w118:errorcluster)  [unwired: 13 in]
    }
    frame "OFDM", Default {
      n41 = call "niDTS WLAN OFDM Tx Test Initialize.vi"("Dut Reference"=w133, "SystemTechnologyCatalog"=w132, "SystemDut"=w131, "Logger Reference"=w134, "error in (no error)"=w136) -> ("OFDM Tx Test Out"=w146:T54, "error out"=w145:errorcluster)  [unwired: 8 in, 1 out]
      n42 = call "niDTS WLAN OFDM Tx Test Configure.vi"("Dummy Test Handle in"=w146, "Cluster"="OFDM Parameters", "ResultsIndex"=w129, "error in (no error)"=w145) -> ("Dummy Test Handle out"=w144:T54, "error out"=w143:errorcluster)  [unwired: 10 in]
      n43 = call "niDTS WLAN OFDM Tx Test UTIL OFDM Parameters to WLAN TX Parameters.vi"("OFDM Parameters"="OFDM Parameters") -> ("WLAN Tx Parameters"=w135:T55)  [unwired: 14 in]
      n44 = call "niDTS WLAN OFDM Tx Test Initiate.vi"("Dummy Test Handle in"=w144, "error in (no error)"=w143) -> ("Dummy Test Handle out"=w142:T54, "error out"=w141:errorcluster)  [unwired: 12 in]
      n45 = call "niDTS WLAN Tx Test UTIL Parameters to DUT Parameters.vi"("Parameters"=w135) -> ("TV Parameters(DataType)"=w148:T59)  [unwired: 14 in]
      n46 = Unbundle By Name(w148) -> ("WLAN Type"=w147:T48)
      n47 = call "niDTS WLAN OFDM Tx Test Fetch Results.vi"("Dummy Test Handle in"=w142, "error in (no error)"=w141) -> ("Dummy Test Handle out"=w140:T54, "Results"=w130:T16, "error out"=w139:errorcluster)  [unwired: 11 in]
      n48 = call "niDTS WLAN OFDM Tx Test Close.vi"("Dummy Test Handle in"=w140, "error in (no error)"=w139) -> ("error out"=w138:errorcluster)  [unwired: 13 in]
    }
    frame "HT" {
      n49 = call "niDTS WLAN HT Tx Test Initialize.vi"("Dut Reference"=w153, "SystemTechnologyCatalog"=w152, "SystemDut"=w151, "Logger Reference"=w154, "error in (no error)"=w159) -> ("Dummy Test Handle out"=w161:T54, "error out"=w162:errorcluster)  [unwired: 8 in, 1 out]
      n50 = call "niDTS WLAN HT Tx Test UTIL HT Parameters to WLAN TX Parameters.vi"("HT Parameters"="HT Parameters") -> ("WLAN Tx Parameters"=w155:T55)  [unwired: 14 in]
      n51 = call "niDTS WLAN HT Tx Test Configure.vi"("Dummy Test Handle in"=w161, "Cluster"="HT Parameters", "ResultsIndex"=w149, "error in (no error)"=w162) -> ("Dummy Test Handle out"=w164:T54, "error out"=w165:errorcluster)  [unwired: 10 in]
      n52 = call "niDTS WLAN Tx Test UTIL Parameters to DUT Parameters.vi"("Parameters"=w155) -> ("TV Parameters(DataType)"=w160:T59)  [unwired: 14 in]
      n53 = call "niDTS WLAN HT Tx Test Initiate.vi"("Dummy Test Handle in"=w164, "error in (no error)"=w165) -> ("Dummy Test Handle out"=w168:T54, "error out"=w163:errorcluster)  [unwired: 12 in]
      n54 = Unbundle By Name(w160) -> ("WLAN Type"=w157:T48)
      n55 = call "niDTS WLAN HT Tx Test Fetch Results.vi"("Dummy Test Handle in"=w168, "error in (no error)"=w163) -> ("Dummy Test Handle out"=w166:T54, "Results"=w150:T16, "error out"=w167:errorcluster)  [unwired: 11 in]
      n56 = call "niDTS WLAN HT Tx Test Close.vi"("Dummy Test Handle in"=w166, "error in (no error)"=w167) -> ("error out"=w156:errorcluster)  [unwired: 13 in]
    }
    frame "VHT" {
      n57 = call "niDTS WLAN VHT Tx Test Initialize.vi"("Dut Reference"=w173, "SystemTechnologyCatalog"=w172, "Specific Socket/Tech DUT Definition"=w171, "Logger Reference"=w175, "error in (no error)"=w182) -> ("Dummy Test Handle out"=w180:T54, "error out"=w185:errorcluster)  [unwired: 8 in, 1 out]
      n58 = call "niDTS WLAN VHT Tx Test Configure.vi"("Dummy Test Handle in"=w180, "Cluster"="VHT Parameters", "ResultsIndex"=w169, "error in (no error)"=w185) -> ("Dummy Test Handle out"=w179:T54, "error out"=w186:errorcluster)  [unwired: 10 in]
      n59 = call "niDTS WLAN VHT Tx Test UTIL VHT Parameters to WLAN TX Parameters.vi"("HT Parameters"="VHT Parameters") -> ("WLAN Tx Parameters"=w174:T55)  [unwired: 14 in]
      n60 = call "niDTS WLAN Tx Test UTIL Parameters to DUT Parameters.vi"("Parameters"=w174) -> ("TV Parameters(DataType)"=w184:T59)  [unwired: 14 in]
      n61 = call "niDTS WLAN VHT Tx Test Initiate.vi"("Dummy Test Handle in"=w179, "error in (no error)"=w186) -> ("Dummy Test Handle out"=w178:T54, "error out"=w188:errorcluster)  [unwired: 12 in]
      n62 = Unbundle By Name(w184) -> ("WLAN Type"=w176:T48)
      n63 = call "niDTS WLAN VHT Tx Test Fetch Results.vi"("Dummy Test Handle in"=w178, "error in (no error)"=w188) -> ("Dummy Test Handle out"=w177:T54, "Results"=w170:T16, "error out"=w187:errorcluster)  [unwired: 11 in]
      n64 = call "niDTS WLAN VHT Tx Test Close.vi"("Dummy Test Handle in"=w177, "error in (no error)"=w187) -> ("error out"=w181:errorcluster)  [unwired: 13 in]
    }
  }
  "Results Type" <- w23
  "Results" <- w9
  "DSSS Results" <- w6
  n65 = flat-sequence {
    tunnel: [w190] -> w5
    tunnel: w21 -> [w194]
    tunnel: w19 -> [w193]
    tunnel: w2 -> [w189]
    tunnel: w12 -> [w191]
    tunnel: [w189] -> w4
    frame #0 {
      # "TestStand Model Plugin Close"
      n66 = flat-sequence {
        tunnel: w194 -> [w197]
        tunnel: [w196] -> w192
        tunnel: w191 -> [w195]
        frame #0 {
          # "Dut Handles Cleanup"
          n67 = call "niDTS TestStand Station Close Dut Handles.vi"("Socket Dut Handles In"=w195, "Close All"=TRUE, "error in (no error)"=w197) -> ("error out"=w196:errorcluster)  [unwired: 11 in, 1 out]
        }
      }
      n68 = call "niDTS TestStand Station Close Instrument Catalog.vi"("Socket Instrument Catalog"=w193, "error in (no error)"=w192) -> ("error out"=w190:errorcluster)  [unwired: 13 in]
    }
  }
  n69 = flat-sequence {
    tunnel: w5 -> [w202]
    tunnel: w4 -> [w200]
    tunnel: [w199] -> w3
    frame #0 {
      # "Close the Logger. Handle Viewer"
      n70 = case shown="True" "Keep Log Open" {
        selector: "Keep Log Open" -> [w205 w207]
        tunnel: w202 -> [w206 w211]
        tunnel: [w206 w211] -> w201
        tunnel: [w205 w207] -> w203
        frame False {
        }
        frame True {
          n71 = property on="Keep Log Open" class="Bool (strict)"("Blinking"=w207) -> (error out=w208:errorcluster)  [unwired: 2 in, 1 out]
          n72 = while {
            tunnel: [w215] -> w209
            tunnel: w208 -> [w214]
            stop <- w213 stop-if-true
            n73 = property on="Keep Log Open" class="Bool (strict)"(error in=w214) -> (error out=w215:errorcluster, "Value"=w212:bool)  [unwired: 1 in, 1 out]
            n74 = Not(x=w212) -> (.not. x?=w213:bool)
            n75 = Wait (ms)(milliseconds to wait=u32 100) -> ()  [unwired: 1 out]
          }
          n76 = property on="Keep Log Open" class="Bool (strict)"(error in=w209, "Blinking"=FALSE) -> ()  [unwired: 1 in, 2 out]
        }
      }
      n77 = property on="Keep Log Open" class="Bool (strict)"("Value"=w203) -> ()  [unwired: 2 in, 2 out]
      n78 = call "niDTS Logger Close.vi"("Logger Handle in"=w200, "error in (no error)"=w201) -> ("error out"=w199:errorcluster)  [unwired: 13 in]
    }
  }
  "error out" <- w3
